vi "good or not to fit.vi"(10 "List Fit Peak In":T1[](array[typedef]), 11 "List ROI In":dbl[][](array[numeric])=[[2.295902819051137, 0.12087567441886224, 747.0, 785.0, 2.233926550867361, 2.356038682169207, 6063.6329279938445, 123.14309366808929], [3.692284511840813, 0.1337148202052189, 1180.0, 1222.0, 3.625362152280503, 3.760328192140438, 67989.42495261344, 852.13028597231], [4.0147483591783155, 0.11975391177237468, 1283.0, 1320.0, 3.956350297651297, 4.075248951813621, 7193.497223633383, 69.57166423918198], [12.573977083982806, 0.2536395480153376, 3925.0, 4004.0, 12.446356900269128, 12.700221594291389, 5812.069028071378, 495.66499136986374]]) -> (2 "List Fit Peak Out":T1[](array[typedef]))   [LabVIEW 2023]
uses:
  control/List Fit peak.ctl
panel:
  in  "R-Sqaure Threshold":dbl=0.2
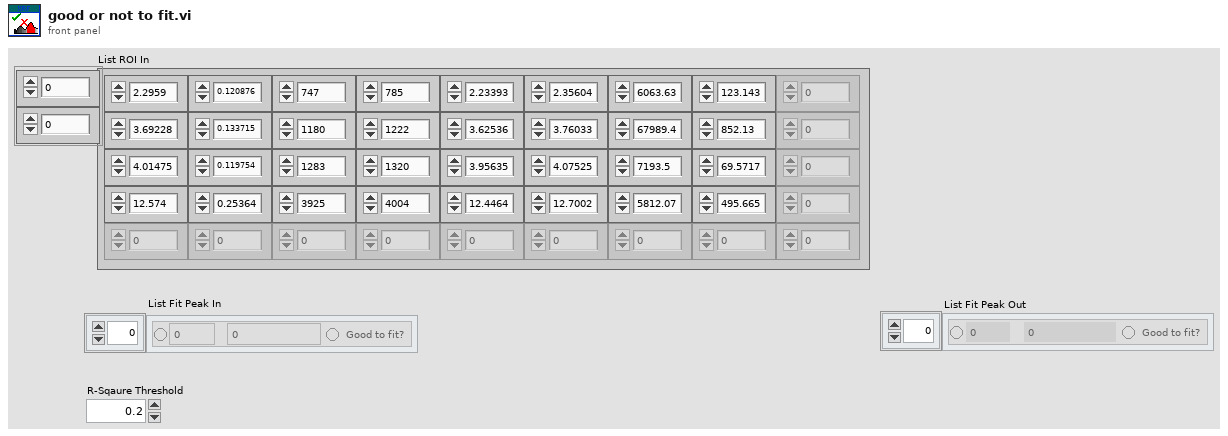
[diagram p1: front panel]
types:
  T1 = typedef "List Fit peak.ctl" = cluster{"Include":bool, "Position":dbl, "Energy":dbl, "good?":bool}
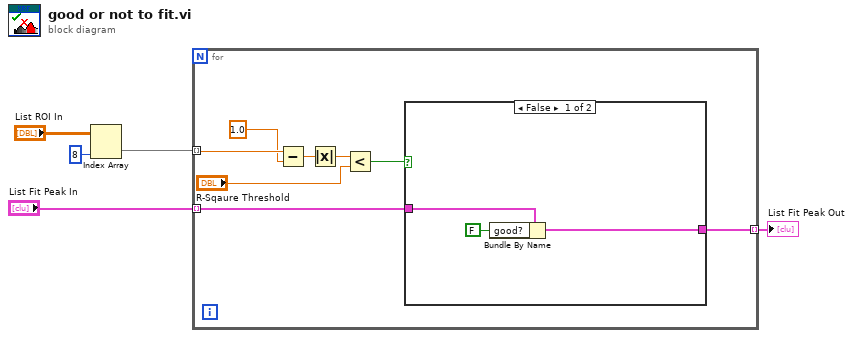
[diagram p0: block diagram]
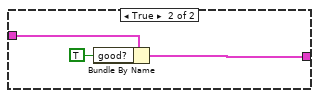
[diagram p2: hidden frame]
diagram:
  n1 = Index Array(array="List ROI In", index (col)=8 ("disabled index (col)")) -> (element=w3:dbl[])  [unwired: 1 in]
  n2 = for {
    tunnel: w3 -> [w13] mode=indexing
    tunnel: "List Fit Peak In" -> [w7] mode=indexing
    tunnel: [w6] -> w1 mode=indexing
    n3 = Subtract(x=w13, y=1.0) -> (x-y=w12:dbl)
    n4 = Absolute Value(x=w12) -> (abs(x)=w11:dbl)
    n5 = Less?(x=w11, y="R-Sqaure Threshold") -> (x < y?=w8:bool)
    n6 = case shown="False" w8 {
      tunnel: w7 -> [w14 w19]
      tunnel: [w15 w17] -> w6
      frame False {
        n7 = Bundle By Name(cluster=w14, "good?"=FALSE) -> (w15:T1)
      }
      frame True {
        n8 = Bundle By Name(cluster=w19, "good?"=TRUE) -> (w17:T1)
      }
    }
  }
  "List Fit Peak Out" <- w1
